vi "Do create project.vi"(8 "error in (no error)":errorcluster, 10 "create_project Argument":T4, 11 "Data Cluster in":T1) -> (0 "error out":errorcluster, 2 "create_project (Reply Payload)":T3, 3 "Data Cluster out":T1)   [LabVIEW 2025, in "Scripting Server.lvlib"]
uses:
  Scripting Server.lvlib
  create_project (Reply Payload)--cluster.ctl
  create_project Argument--cluster.ctl
  Config Data.ctl
  Module Data--cluster.ctl
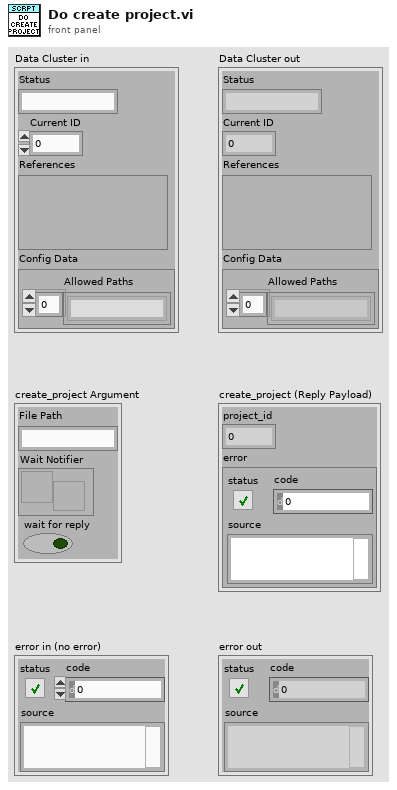
[diagram p1: front panel]
types:
  T1 = typedef "Scripting Server.lvlib/Module Data--cluster.ctl" = cluster{"Status":string, "Current ID":i32, "References":variant, "Config Data":T2}
  T2 = typedef "Scripting Server.lvlib/Config Data.ctl" = cluster{"Allowed Paths":string[]}
  T3 = typedef "Scripting Server.lvlib/create_project (Reply Payload)--cluster.ctl" = cluster{"project_id":i32, "error":errorcluster}
  T4 = typedef "Scripting Server.lvlib/create_project Argument--cluster.ctl" = cluster{"File Path":string, "Wait Notifier":refnum<notifier>, "wait for reply":bool}
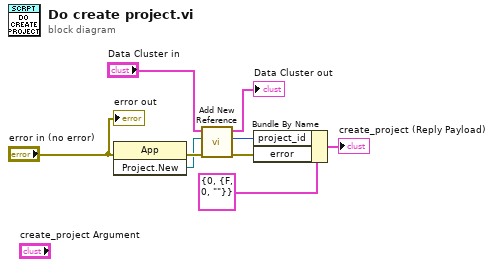
[diagram p0: block diagram]
diagram:
  n1 = invoke class="App" method="Project.New"(error in="error in (no error)") -> (error out=w5:errorcluster, "Project:New"=w2:refnum<vi>)  [unwired: 2 in, 1 out]
  n2 = call "Add New Reference.vi"("error in (no error)"=w5, "Variant"=w2, "Data Cluster in"="Data Cluster in") -> ("error out"=w4:errorcluster, "new reference"=w1:i32, "Data Cluster out 2"=→"Data Cluster out":T1)  [unwired: 6 in]
  n3 = Bundle By Name(cluster=T3 {"project_id"=0, "error"={"status"=FALSE, "code"=0, "source"=""}} ("create_project (Reply Payload)"), "project_id"=w1, "error"=w4) -> (→"create_project (Reply Payload)":T3)
  "error out" <- "error in (no error)"
